vi "Jacobian Elliptic Functions.vi"(6 "k":dbl format="%.2f", 7 "x":dbl format="%.2f") -> (0 "phi":dbl format="%.2f", 1 "sn":dbl format="%.2f", 2 "dn":dbl format="%.2f", 3 "cn":dbl format="%.2f")   [LabVIEW 2017, in "NI_Gmath.lvlib"]
doc: "Determines the Jacobian elliptic functions <B>cn</B>, <B>dn</B>, and <B>sn</B>."
uses:
  <vilib>/gmath/NI_Gmath.lvlib
  <resource>/lvanlys.dll
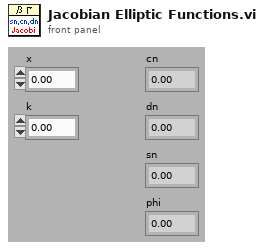
[diagram p1: front panel]
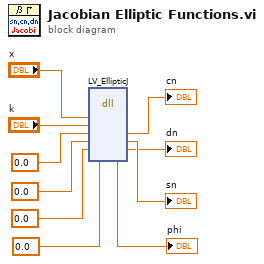
[diagram p0: block diagram]
diagram:
  n1 = dll-call lib="e:/builds/penguin/labview/branches/2017/dev/dist/resource/lvanlys.*" fn="LV_EllipticJ"("x"="x", "k"="k", "cn"=0.0, "sn"=0.0, "dn"=0.0, "phi"=0.0) -> ("cn"=→"cn":dbl, "sn"=→"sn":dbl, "dn"=→"dn":dbl, "phi"=→"phi":dbl)  [unwired: 6 in, 2 out]
